vi "DAQ-WriteValue.vi"(6 "Input":dbl format="%0.2f", 7 "Limites":T2, 8 "DAQ?":bool, 9 "DAQ Device IN":T1={"DAQ Fs (S/s)"=10000.0, "task"="", "error"={"status"=FALSE, "code"=0, "source"=""}, "Min Value"=-10.0, "Max Value"=10.0}) -> (3 "DAQ Device OUT":T1={"DAQ Fs (S/s)"=0.0, "task"="", "error"={"status"=FALSE, "code"=0, "source"=""}, "Min Value"=-10.0, "Max Value"=10.0})   [LabVIEW 2010]
uses:
  <vilib>/DAQmx/write.llb/DAQmx Write (Analog DBL 1Chan 1Samp).vi
  <vilib>/daqmx/miscellaneous.llb/DAQmx Fill In Error Info.vi
panel:
  out "#samples out":u32
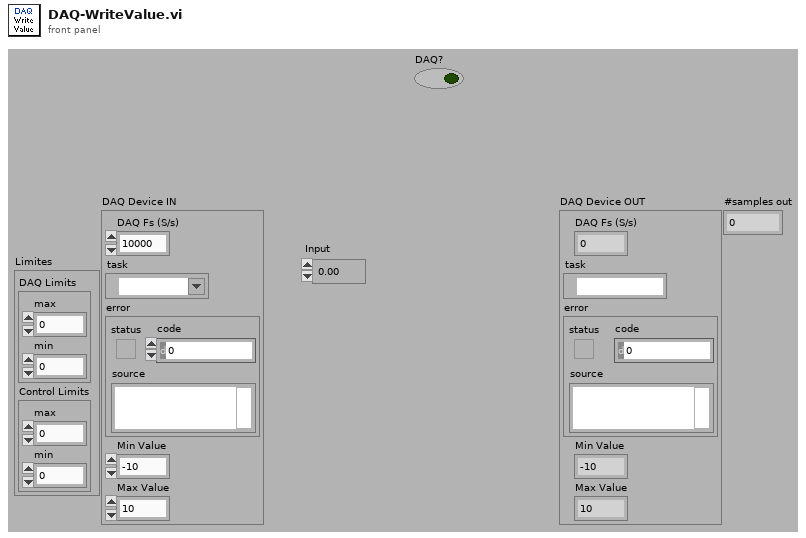
[diagram p1: front panel]
types:
  T1 = cluster{"DAQ Fs (S/s)":dbl, "task":refnum<k21>, "error":errorcluster, "Min Value":dbl, "Max Value":dbl}
  T2 = cluster{"DAQ Limits":cluster{"max":dbl, "min":dbl}, "Control Limits":cluster{"max":dbl, "min":dbl}}
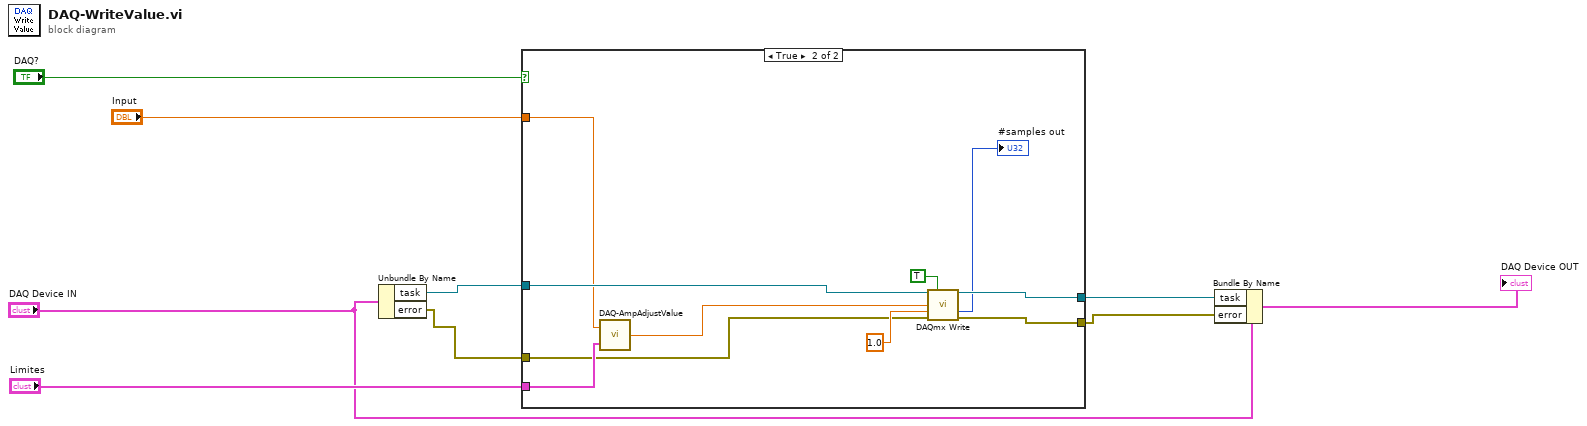
[diagram p0: block diagram]
diagram:
  n1 = Unbundle By Name("DAQ Device IN") -> ("task"=w5:refnum<k21>, "error"=w1:errorcluster)
  n2 = case shown="True" "DAQ?" {
    tunnel: w5 -> [w10 w15]
    tunnel: [w10 w20] -> w3
    tunnel: w1 -> [w11 w14]
    tunnel: [w11 w19] -> w4
    tunnel: "Limites" -> [_ w21]
    tunnel: "Input" -> [_ w13]
    frame False {
    }
    frame True {
      n3 = call "DAQ-AmpAdjustValue.vi"("Limites"=w21, "Input"=w13) -> ("Output"=w12:dbl)
      n4 = call-poly <vilib>:"DAQmx Write.vi"("task/channels in"=w15, "auto start"=TRUE, "data"=w12, "timeout"=1.0, "error in"=w14) -> ("task out"=w20:refnum<k21>, "number of samples written per channel"=→"#samples out":u32, "error out"=w19:errorcluster)  [unwired: 8 in]
    }
  }
  n5 = Bundle By Name(cluster="DAQ Device IN", "task"=w3, "error"=w4) -> (→"DAQ Device OUT":T1)
